vi "ff close.vi"() -> (3 "function return":i32)   [LabVIEW 2013, in "ffvi.lvlib"]
doc: "int ff_close();"
uses:
  ffvi.lvlib
  ffvi.dll
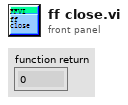
[diagram p1: front panel]
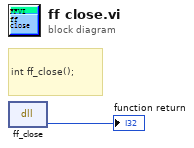
[diagram p0: block diagram]
diagram:
  # "int ff_close();"
  n1 = dll-call lib="D:/ffmpeg/ffvi/ffvi.*" fn="ff_close"() -> ("return type"=→"function return":i32)  [unwired: 3 in, 2 out]
